vi "New TDMS Sink.vi"(8 "error in (no error)":errorcluster, 11 "TDMS File Path":path) -> (0 "error out":errorcluster, 3 "TDMS out":refnum<class "TDMS Sink.lvclass">)   [LabVIEW 2020, in "LV Log.lvlib" / "TDMS Sink.lvclass"]
uses:
  TDMS Sink.lvclass
  TDMS Sink.lvclass/TDMS Sink.ctl
panel:
  in  "Group Name":string
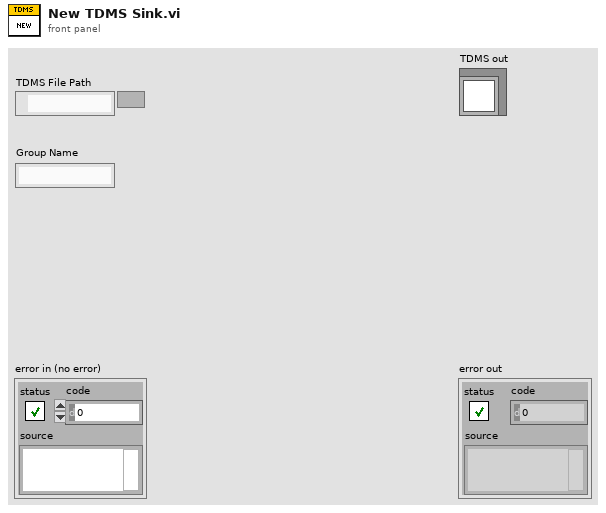
[diagram p1: front panel]
types:
  T1 = enum16{"open", "open or create", "create or replace", "create", "open (read-only)"}
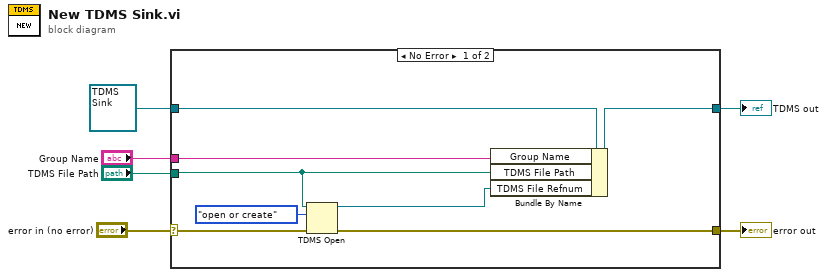
[diagram p0: block diagram]
diagram:
  n1 = case shown="No Error" "error in (no error)" {
    selector: "error in (no error)" -> [w12 w16]
    tunnel: [w11 w16] -> w5
    tunnel: [w13 w15] -> w3
    tunnel: refnum<class "TDMS Sink.lvclass"> refnum ("TDMS in") -> [w14 w15]
    tunnel: "TDMS File Path" -> [w10 _]
    tunnel: "Group Name" -> [w7 _]
    frame No Error {
      n2 = TDMS Open(8:w12, 10:T1."open or create" ("operation (0:open)"), 11:w10) -> (0:w11:errorcluster, 3:w8:refnum<k34>)  [unwired: 4 in]
      n3 = Bundle By Name(cluster=w14, "Group Name"=w7, "TDMS File Path"=w10, "TDMS File Refnum"=w8) -> (w13:refnum<class "TDMS Sink.lvclass">)
    }
    frame Error {
    }
  }
  "error out" <- w5
  "TDMS out" <- w3
